vi "ExcelReport.vi"(6 "SN":string="1", 8 "error in":errorcluster caption="错误输入（无错误）", 10 "列首字符串":string[](array[string])=["测试名称", "TestItem ITEM", "通道", "设置参数", "下限值", "上限值", "单位", "测量值", "结果", "测试时间", "备注", "测试项目"], 11 "TestResults":string[][](table)=[["启动测试程序", "CMD", "启动测试程序", "100", "", "", "", "PASS", "PASS", "27.534000", "", "通信", "0"], ["测量电流", "MeaCurrent", "Current", "Differential", "0.65", "1", "A", "0.75051", "PASS", "1.079000", "", "电流", "0"], ["启动蓝牙模块", "CMD", "启动蓝牙模块", "1000", "", "", "Hex", "PASS", "PASS", "1.065000", "", "蓝牙", "0"], ["延时", "Delay", "", "2", "", "", "s", "", "Done", "2.023000", "延时2s", "蓝牙", "0"], ["蓝牙状态查询", "CMD", "蓝牙状态查询", "1000", "0x00", "0x00", "Hex", "0x00", "PASS", "5.294000", "", "蓝牙", "1"], ["打开蓝牙", "CMD", "蓝牙打开", "100", "0x00", "0x00", "Hex", "0x00", "PASS", "0.185000", "", "蓝牙", "0"], ["设置音量20", "CMD", "设置系统音量20", "100", "0x00", "0x00", "Hex", "0x00", "PASS", "0.189000", "", "通信", "0"], ["启动屏幕校准", "CMD", "启动屏幕校准", "100", "", "", "Hex", "PASS", "PASS", "0.189000", "", "屏幕校准", "0"], ["人工校准屏幕", "Check", "屏幕校准", "VisualCheck.vi", "", "", "", "PASS", "PASS", "11.176000", "", "屏幕校准", "0"], ["启动按键测试", "CMD", "启动按键模块", "100", "", "", "Hex", "PASS", "PASS", "0.169000", "", "按键", "0"], ["按键测试", "Check", "按键", "VisualCheck.vi", "", "", "", "PASS", "PASS", "11.933000", "", "按键", "0"], ["退出按键测试", "CMD", "按键模块退出", "100", "", "", "Hex", "PASS", "PASS", "0.171000", "", "按键", "0"], ["DVD仓口灯光", "Check", "DVD灯光蓝色", "VisualCheck.vi", "", "", "", "PASS", "PASS", "4.402000", "", "DVD", "0"], ["入碟", "Check", "放入CD碟", "VisualCheck.vi", "", "", "", "PASS", "PASS", "6.804000", "", "DVD", "0"], ["DVD仓口灯光", "Check", "DVD灯光红色", "VisualCheck.vi", "", "", "", "PASS", "PASS", "2.171000", "", "DVD", "0"], ["打开ILL", "DOAction", "ILL", "1", "", "", "电平", "", "Done", "0.013000", "", "ILL检测", "0"], ["按键灯", "Check", "按键灯亮", "VisualCheck.vi", "", "", "", "PASS", "PASS", "1.676000", "", "按键", "0"], ["读取ILL状态", "CMD", "ILL状态", "100", "0x01", "0x01", "Hex", "0x01", "PASS", "0.170000", "", "ILL检测", "0"], ["关闭ILL", "DOAction", "ILL", "0", "", "", "电平", "", "Done", "0.013000", "", "ILL检测", "0"], ["打开BACK", "DOAction", "BACK", "1", "", "", "电平", "", "Done", "0.013000", "", "倒车检测", "0"], ["倒车视频", "Check", "倒车视频", "VisualCheck.vi", "", "", "", "PASS", "PASS", "1.476000", "", "倒车检测", "0"], ["读取BACK状态", "CMD", "BACK状态", "100", "0x01", "0x01", "Hex", "0x01", "PASS", "0.169000", "", "倒车检测", "0"], ["关闭BACK", "DOAction", "BACK", "0", "", "", "电平", "", "Done", "0.013000", "", "倒车检测", "0"], ["打开BREAK", "DOAction", "BRAKE", "1", "", "", "电平", "", "Done", "0.013000", "", "刹车检测", "0"], ["延时", "Delay", "", "0.5", "", "", "s", "", "Done", "0.512000", "延时500ms", "刹车检测", "0"], ["读取BREAK状态", "CMD", "BRAKE状态", "100", "0x01", "0x01", "Hex", "0x01", "PASS", "0.190000", "", "刹车检测", "0"], ["关闭BREAK", "DOAction", "BRAKE", "0", "", "", "电平", "", "Done", "0.030000", "", "刹车检测", "0"], ["启动方控模块", "CMD", "启动方控模块", "100", "", "", "Hex", "PASS", "PASS", "0.189000", "", "方控", "0"], ["打开方控1输出", "DOAction", "SW1", "1", "", "", "电平", "", "Done", "0.032000", "", "方控", "0"], ["读取方控1电压值", "CMD", "读取SW1电压", "200", "2.2", "2.5", "Hex", "3.26697", "FAIL", "2.297000", "方控1,2~2.2V", "方控", "0"], ["关闭方控1输出", "DOAction", "SW1", "0", "", "", "电平", "", "Done", "0.030000", "", "方控", "0"], ["打开方控2输出", "DOAction", "SW2", "1", "", "", "电平", "", "Done", "0.030000", "", "方控", "0"], ["读取方控1电压值", "CMD", "读取SW2电压", "100", "2.2", "2.5", "Hex", "3.26858", "FAIL", "1.362000", "方控2,2~2.2V", "方控", "0"], ["关闭方控2输出", "DOAction", "SW2", "0", "", "", "电平", "", "Done", "0.030000", "", "方控", "0"], ["获取蓝牙地址", "CMD", "获取蓝牙地址", "500", "0x000000000000", "0xFFFFFFFFFFFF", "Hex", "0x882020202020", "PASS", "2.216000", "", "蓝牙", "1"], ["延时", "Delay", "", "1", "", "", "s", "", "Done", "1.028000", "延时1s", "蓝牙", "0"], ["蓝牙配对", "CMD", "蓝牙配对", "500", "0x00", "0x00", "Hex", "0x00", "PASS", "3.089000", "", "蓝牙", "1"], ["蓝牙状态查询", "CMD", "蓝牙状态查询", "100", "0x06", "0x06", "Hex", "0x06", "PASS", "0.201000", "", "蓝牙", "1"], ["打开喇叭输出", "DOAction", "SPK", "1", "", "", "电平", "", "Done", "0.043000", "", "蓝牙", "0"], ["延时", "Delay", "", "1", "", "", "s", "", "Done", "1.023000", "延时1s", "蓝牙", "0"], ["音频模拟输出", "AOFreq", "AudioSW", "F=1000HZ,A=0.6V", "", "", "频率", "", "Done", "1.230000", "", "蓝牙", "0"], ["采集蓝牙音频输出", "BlueToothAI", "", "", "", "", "", "", "Done", "4.457000", "", "蓝牙", "0"], ["蓝牙音频频率", "Frequency", "", "", "980", "1020", "Hz", "909.76991", "FAIL", "0.025000", "", "蓝牙", "0"], ["蓝牙音频幅度", "RMS", "", "", "0.2", "0.5", "V", "0.00002", "FAIL", "0.013000", "", "蓝牙", "0"], ["蓝牙音频失真度", "BTTHD", "", "", "0", "1", "%", "100.65435", "FAIL", "0.034000", "", "蓝牙", "0"], ["关闭喇叭输出", "DOAction", "SPK", "0", "", "", "电平", "", "Done", "0.012000", "", "蓝牙", "0"], ["关闭音频模拟输出", "AOFreq", "AudioSW", "F=0HZ,A=0V", "", "", "频率", "", "Done", "1.013000", "", "蓝牙", "0"], ["关闭蓝牙", "CMD", "蓝牙关闭", "500", "0x00", "0x00", "Hex", "0x00", "PASS", "1.596000", "", "蓝牙", "0"], ["退出蓝牙模块", "CMD", "蓝牙模块退出", "100", "", "", "Hex", "PASS", "PASS", "0.539000", "", "蓝牙", "0"], ["清除蓝牙设备", "RemoveBTDevices", "", "", "", "", "", "", "Done", "0.656000", "", "", "0"], ["检测SD卡", "CMD", "SD卡状态", "100", "0x01", "0x01", "Hex", "0x01", "PASS", "0.172000", "", "SD卡", "1"], ["启动SD卡模块", "CMD", "启动SD卡模块", "500", "", "", "Hex", "PASS", "PASS", "3.664000", "", "SD卡", "1"], ["SD卡加载状态", "CMD", "SD卡加载状态", "100", "0x02", "0x02", "Hex", "0x02", "PASS", "0.176000", "", "SD卡", "1"], ["SD卡加载时间", "CMD", "SD卡加载时间", "100", "0", "10", "s", "0.00000", "PASS", "0.273000", "0~10s加载时间", "SD卡", "0"], ["播放SD卡音频2", "CMD", "播放SD卡音频2", "100", "0x00", "0x00", "Hex", "0x00", "PASS", "2.141000", "", "SD卡", "0"], ["延时", "Delay", "", "1", "", "", "s", "", "Done", "1.029000", "延时1s", "SD卡", "0"], ["采集FL音频输出", "AIFreq", "FL", "Differential", "", "", "", "", "Done", "1.037000", "", "SD卡", "0"], ["FL频率", "Frequency", "", "", "990", "1010", "Hz", "999.96860", "PASS", "0.034000", "", "SD卡", "0"], ["FL幅度", "RMS", "", "", "0.9", "1.1", "V", "0.96949", "PASS", "0.016000", "", "SD卡", "0"], ["FL失真度", "THD", "", "", "0", "1", "%", "0.35018", "PASS", "0.065000", "", "SD卡", "0"], ["采集FR音频输出", "AIFreq", "FR", "Differential", "", "", "", "", "Done", "1.019000", "", "SD卡", "0"], ["FR频率", "Frequency", "", "", "990", "1010", "Hz", "999.96849", "PASS", "0.025000", "", "SD卡", "0"], ["FR幅度", "RMS", "", "", "0.9", "1.1", "V", "0.98085", "PASS", "0.014000", "", "SD卡", "0"], ["FR失真度", "THD", "", "", "0", "1", "%", "0.33911", "PASS", "0.044000", "", "SD卡", "0"], ["采集RL音频输出", "AIFreq", "RL", "Differential", "", "", "", "", "Done", "1.018000", "", "SD卡", "0"], ["RL频率", "Frequency", "", "", "990", "1010", "Hz", "999.96854", "PASS", "0.023000", "", "SD卡", "0"], ["RL幅度", "RMS", "", "", "0.9", "1.1", "V", "0.93852", "PASS", "0.015000", "", "SD卡", "0"], ["RL失真度", "THD", "", "", "0", "1", "%", "0.34994", "PASS", "0.051000", "", "SD卡", "0"], ["采集RR音频输出", "AIFreq", "RR", "Differential", "", "", "", "", "Done", "1.020000", "", "SD卡", "0"], ["RR频率", "Frequency", "", "", "990", "1010", "Hz", "999.96869", "PASS", "0.026000", "", "SD卡", "0"], ["RR幅度", "RMS", "", "", "0.9", "1.1", "V", "0.93560", "PASS", "0.014000", "", "SD卡", "0"], ["RR失真度", "THD", "", "", "0", "1", "%", "0.35691", "PASS", "0.051000", "", "SD卡", "0"], ["采集FLOUT音频输出", "AIFreq", "FLOUT", "RSE", "", "", "", "", "Done", "1.018000", "", "SD卡", "0"], ["FLOUT频率", "Frequency", "", "", "990", "1010", "Hz", "999.96842", "PASS", "0.023000", "", "SD卡", "0"], ["FLOUT幅度", "RMS", "", "", "0.09", "0.11", "V", "0.04812", "FAIL", "0.014000", "", "SD卡", "0"], ["采集FROUT音频输出", "AIFreq", "FROUT", "RSE", "", "", "", "", "Done", "1.019000", "", "SD卡", "0"], ["FROUT频率", "Frequency", "", "", "990", "1010", "Hz", "999.96823", "PASS", "0.024000", "", "SD卡", "0"], ["FROUT幅度", "RMS", "", "", "0.09", "0.11", "V", "0.04856", "FAIL", "0.014000", "", "SD卡", "0"], ["采集RLOUT音频输出", "AIFreq", "RLOUT", "RSE", "", "", "", "", "Done", "1.020000", "", "SD卡", "0"], ["RLOUT频率", "Frequency", "", "", "990", "1010", "Hz", "999.96809", "PASS", "0.024000", "", "SD卡", "0"], ["RLOUT幅度", "RMS", "", "", "0.09", "0.11", "V", "0.04613", "FAIL", "0.015000", "", "SD卡", "0"], ["采集RROUT音频输出", "AIFreq", "RROUT", "RSE", "", "", "", "", "Done", "1.018000", "", "SD卡", "0"], ["RROUT频率", "Frequency", "", "", "990", "1010", "Hz", "999.96763", "PASS", "0.025000", "", "SD卡", "0"], ["RROUT幅度", "RMS", "", "", "0.09", "0.11", "V", "0.04594", "FAIL", "0.014000", "", "SD卡", "0"], ["播放SD卡音频7", "CMD", "播放SD卡音频7", "100", "0x00", "0x00", "Hex", "0x00", "PASS", "0.425000", "", "SD卡", "0"], ["延时", "Delay", "", "1", "", "", "s", "", "Done", "1.013000", "延时1s", "SD卡", "0"], ["采集FL音频输出", "AIFreq", "FL", "Differential", "", "", "", "", "Done", "1.039000", "", "SD卡", "0"], ["FL信噪比", "SNR", "", "", "45", "", "db", "53.79027", "PASS", "0.015000", "", "SD卡", "0"], ["采集FR音频输出", "AIFreq", "FR", "Differential", "", "", "", "", "Done", "1.019000", "", "SD卡", "0"], ["FR信噪比", "SNR", "", "", "45", "", "db", "53.09428", "PASS", "0.015000", "", "SD卡", "0"], ["采集RL音频输出", "AIFreq", "RL", "Differential", "", "", "", "", "Done", "1.017000", "", "SD卡", "0"], ["RL信噪比", "SNR", "", "", "45", "", "db", "52.88284", "PASS", "0.014000", "", "SD卡", "0"], ["采集RR音频输出", "AIFreq", "RR", "Differential", "", "", "", "", "Done", "1.018000", "", "SD卡", "0"], ["RR信噪比", "SNR", "", "", "45", "", "db", "53.42465", "PASS", "0.013000", "", "SD卡", "0"], ["播放SD卡音频8", "CMD", "播放SD卡音频8", "100", "0x00", "0x00", "Hex", "0x00", "PASS", "0.425000", "", "SD卡", "0"], ["延时", "Delay", "", "1", "", "", "s", "", "Done", "1.013000", "延时1s", "SD卡", "0"], ["采集FL音频输出", "AIsFreq", "CH1=FL,CH2=FR", "Differential", "", "", "", "", "Done", "1.037000", "", "SD卡", "0"], ["FL分离度", "crosstalk", "", "", "45", "", "db", "52.77644", "PASS", "0.036000", "", "SD卡", "0"], ["采集RL音频输出", "AIsFreq", "CH1=RL,CH2=RR", "Differential", "", "", "", "", "Done", "1.020000", "", "SD卡", "0"], ["RL分离度", "crosstalk", "", "", "45", "", "db", "51.94792", "PASS", "0.032000", "", "SD卡", "0"], ["播放SD卡音频10", "CMD", "播放SD卡音频10", "100", "0x00", "0x00", "Hex", "0x00", "PASS", "0.432000", "", "SD卡", "0"], ["延时", "Delay", "", "1", "", "", "s", "", "Done", "1.013000", "延时1s", "SD卡", "0"], ["采集FR音频输出", "AIsFreq", "CH1=FR,CH2=FL", "Differential", "", "", "", "", "Done", "1.037000", "", "SD卡", "0"], ["FR分离度", "crosstalk", "", "", "45", "", "db", "52.76491", "PASS", "0.034000", "", "SD卡", "0"], ["采集RR音频输出", "AIsFreq", "CH1=RR,CH2=RL", "Differential", "", "", "", "", "Done", "1.019000", "", "SD卡", "0"], ["RR分离度", "crosstalk", "", "", "45", "", "db", "51.83152", "PASS", "0.034000", "", "SD卡", "0"], ["退出SD卡模块", "CMD", "SD卡模块退出", "100", "", "", "Hex", "PASS", "PASS", "0.486000", "", "SD卡", "0"], ["检测USB", "CMD", "USB状态", "100", "0x01", "0x01", "Hex", "0x00", "FAIL", "3.035000", "", "USB", "1"], ["启动USB模块", "CMD", "启动USB模块", "500", "", "", "Hex", "", "Skip", "0.032000", "", "USB", "1"], ["USB加载状态", "CMD", "USB加载状态", "100", "0x02", "0x02", "Hex", "", "Skip", "0.020000", "", "USB", "0"], ["USB加载时间", "CMD", "USB加载时间", "100", "0", "10", "s", "", "Skip", "0.012000", "1~10s加载时间", "USB", "0"], ["退出USB模块", "CMD", "USB模块退出", "100", "", "", "Hex", "", "Skip", "0.013000", "", "USB", "0"], ["设置音量20", "CMD", "设置系统音量20", "100", "0x00", "0x00", "Hex", "0x00", "PASS", "0.174000", "", "通信", "0"], ["IPOD_DET下拉", "DOAction", "IPOD_DET", "1", "", "", "电平", "", "Done", "0.015000", "", "IPOD", "0"], ["延时", "Delay", "", "0.5", "", "", "s", "", "Done", "0.514000", "延时0.5s", "IPOD", "0"], ["启动IPOD模块", "CMD", "启动IPOD", "500", "", "", "Hex", "PASS", "PASS", "2.413000", "", "IPOD", "1"], ["IPOD通信测试", "CMD", "IPOD通信自检", "100", "0x00", "0x00", "Hex", "0x00", "PASS", "0.498000", "", "IPOD", "0"], ["打开IPOD电压通道", "DOAction", "DO_IPOD+5V", "1", "", "", "电平", "", "Done", "0.033000", "", "IPOD", "0"], ["IPOD+5V检测", "AIVolt", "IPOD+5V", "", "4.8", "5.5", "V", "5.30354", "PASS", "0.141000", "", "IPOD", "0"], ["关闭IPOD电压通道", "DOAction", "DO_IPOD+5V", "0", "", "", "电平", "", "Done", "0.014000", "", "IPOD", "0"], ["打开IPOD音频通道", "DOAction", "LineOut1", "1", "", "", "电平", "", "Done", "0.015000", "", "IPOD", "0"], ["音频模拟输出", "AOFreq", "AudioSW", "F=1000HZ,A=1V", "", "", "频率", "", "Done", "1.114000", "", "IPOD", "0"], ["采集音频输出", "AIFreq", "FL", "Differential", "", "", "", "", "Done", "1.040000", "", "IPOD", "0"], ["频率", "Frequency", "", "", "990", "1010", "Hz", "1000.00001", "PASS", "0.025000", "", "IPOD", "0"], ["幅度", "RMS", "", "", "0.9", "1.2", "V", "1.06999", "PASS", "0.014000", "", "IPOD", "0"], ["失真度", "THD", "", "", "0", "1", "%", "0.28079", "PASS", "0.047000", "", "IPOD", "0"], ["关闭音频模拟输出", "AOFreq", "AudioSW", "F=0HZ,A=0V", "", "", "频率", "", "Done", "1.015000", "", "IPOD", "0"], ["关闭IPOD音频通道", "DOAction", "LineOut1", "0", "", "", "电平", "", "Done", "0.033000", "", "IPOD", "0"], ["退出IPOD", "CMD", "IPOD退出", "100", "", "", "Hex", "PASS", "PASS", "0.241000", "", "IPOD", "0"], ["启动终端模块", "CMD", "启动TN", "500", "", "", "Hex", "PASS", "PASS", "0.562000", "", "终端", "0"], ["终端通信测试", "CMD", "TN通信自检", "500", "0x00", "0x00", "Hex", "0x00", "PASS", "0.561000", "", "终端", "0"], ["设置TN音量31", "CMD", "设置TN音量31", "100", "0x00", "0x00", "Hex", "0x00", "PASS", "0.166000", "", "终端", "0"], ["打开终端音频通道", "DOAction", "LineOut2", "1", "0x00", "0x00", "电平", "", "Done", "0.004000", "", "终端", "0"], ["音频模拟输出", "AOFreq", "AudioSW", "F=1000HZ,A=1V", "", "", "频率", "", "Done", "1.102000", "", "终端", "0"], ["采集音频输出", "AIFreq", "FL", "Differential", "", "", "", "", "Done", "1.042000", "", "终端", "0"], ["频率", "Frequency", "", "", "990", "1010", "Hz", "1000.00004", "PASS", "0.025000", "", "终端", "0"], ["幅度", "RMS", "", "", "0.9", "1.2", "V", "1.05423", "PASS", "0.017000", "", "终端", "0"], ["失真度", "THD", "", "", "0", "1", "%", "0.31067", "PASS", "0.040000", "", "终端", "0"], ["关闭音频模拟输出", "AOFreq", "AudioSW", "F=0HZ,A=0V", "", "", "频率", "", "Done", "1.014000", "", "终端", "0"], ["关闭终端音频通道", "DOAction", "LineOut2", "0", "", "", "电平", "", "Done", "0.034000", "", "终端", "0"], ["退出终端", "CMD", "TN退出", "100", "", "", "Hex", "PASS", "PASS", "0.183000", "", "终端", "0"], ["启动数字电视模块", "CMD", "启动数字电视", "500", "", "", "Hex", "PASS", "PASS", "6.766000", "", "数字电视", "0"], ["数字电视通信测试", "CMD", "数字电视通信自检", "100", "0x00", "0x00", "Hex", "0x00", "PASS", "0.497000", "", "数字电视", "0"], ["打开DTV音频通道", "DOAction", "LineOut3", "1", "", "", "电平", "", "Done", "0.034000", "", "数字电视", "0"], ["音频模拟输出", "AOFreq", "AudioSW", "F=1000HZ,A=1V", "", "", "频率", "", "Done", "1.119000", "", "数字电视", "0"], ["采集音频输出", "AIFreq", "FL", "Differential", "", "", "", "", "Done", "1.040000", "", "数字电视", "0"], ["频率", "Frequency", "", "", "990", "1010", "Hz", "1000.00015", "PASS", "0.026000", "", "数字电视", "0"], ["幅度", "RMS", "", "", "0.9", "1.2", "V", "1.07136", "PASS", "0.014000", "", "数字电视", "0"], ["失真度", "THD", "", "", "0", "1", "%", "0.31151", "PASS", "0.048000", "", "数字电视", "0"], ["关闭音频模拟输出", "AOFreq", "AudioSW", "F=0HZ,A=0V", "", "", "频率", "", "Done", "1.014000", "", "数字电视", "0"], ["关闭终端音频通道", "DOAction", "LineOut3", "0", "", "", "电平", "", "Done", "0.035000", "", "数字电视", "0"], ["检测视频输出", "Check", "视频播放", "VisualCheck.vi", "", "", "", "PASS", "PASS", "2.188000", "", "数字电视", "0"], ["退出数字电视", "CMD", "数字电视退出", "100", "", "", "Hex", "PASS", "PASS", "0.323000", "", "数字电视", "0"], ["启动AUXIN模块", "CMD", "启动AUXIN", "500", "", "", "Hex", "PASS", "PASS", "3.662000", "", "AuxIn", "0"], ["打开AUXIN音频通道", "DOAction", "LineOut4", "1", "", "", "电平", "", "Done", "0.036000", "", "AuxIn", "0"], ["音频模拟输出", "AOFreq", "AudioSW", "F=1000HZ,A=1V", "", "", "频率", "", "Done", "1.116000", "", "AuxIn", "0"], ["采集音频输出", "AIFreq", "FL", "Differential", "", "", "", "", "Done", "1.040000", "", "AuxIn", "0"], ["频率", "Frequency", "", "", "990", "1010", "Hz", "1000.00011", "PASS", "0.025000", "", "AuxIn", "0"], ["幅度", "RMS", "", "", "0.9", "1.2", "V", "1.04477", "PASS", "0.014000", "", "AuxIn", "0"], ["失真度", "THD", "", "", "0", "1", "%", "0.30972", "PASS", "0.046000", "", "AuxIn", "0"], ["关闭音频模拟输出", "AOFreq", "AudioSW", "F=0HZ,A=0V", "", "", "频率", "", "Done", "1.015000", "", "AuxIn", "0"], ["关闭终端音频通道", "DOAction", "LineOut4", "0", "", "", "电平", "", "Done", "0.036000", "", "AuxIn", "0"], ["检测视频输出", "Check", "视频播放", "VisualCheck.vi", "", "", "", "PASS", "PASS", "1.386000", "", "AuxIn", "0"], ["退出AUXIN", "CMD", "AUXIN退出", "100", "", "", "Hex", "PASS", "PASS", "0.322000", "", "AuxIn", "0"], ["检测DVD状态", "CMD", "DVD碟片状态", "100", "0x01", "0x01", "Hex", "0x01", "PASS", "0.174000", "", "DVD", "1"], ["启动DVD模块", "CMD", "启动DVD模块", "1000", "", "", "", "PASS", "PASS", "2.408000", "", "DVD", "1"], ["等待读碟", "Check", "等待读碟", "VisualCheck.vi", "", "", "", "PASS", "PASS", "14.299000", "", "DVD", "0"], ["DVD加载状态", "CMD", "DVD加载状态", "100", "0x02", "0x02", "Hex", "0x02", "PASS", "0.882000", "", "DVD", "1"], ["DVD加载时间", "CMD", "DVD加载时间", "100", "5", "20", "s", "13.00000", "PASS", "0.198000", "5~20秒加载时间", "DVD", "0"], ["DVD碟片类型", "CMD", "DVD碟片类型", "100", "0x03", "0x03", "Hex", "0x03", "PASS", "1.759000", "CD碟", "DVD", "1"], ["播放DVD曲目2", "CMD", "播放DVD音频2", "100", "0x00", "0x00", "Hex", "0x00", "PASS", "0.548000", "1V 0dB音频", "DVD", "0"], ["延时", "Delay", "", "1", "", "", "s", "", "Done", "1.035000", "延时2s", "DVD", "0"], ["采集FL音频输出", "AIFreq", "FL", "Differential", "", "", "", "", "Done", "1.044000", "", "DVD", "0"], ["FL频率", "Frequency", "", "", "990", "1010", "Hz", "999.96399", "PASS", "0.026000", "", "DVD", "0"], ["FL幅度", "RMS", "", "", "0.9", "1.1", "V", "0.97179", "PASS", "0.016000", "", "DVD", "0"], ["FL失真度", "THD", "", "", "0", "1", "%", "0.61446", "PASS", "0.053000", "", "DVD", "0"], ["采集FR音频输出", "AIFreq", "FR", "Differential", "", "", "", "", "Done", "1.019000", "", "DVD", "0"], ["FR频率", "Frequency", "", "", "990", "1010", "Hz", "999.96393", "PASS", "0.027000", "", "DVD", "0"], ["FR幅度", "RMS", "", "", "0.9", "1.1", "V", "0.98312", "PASS", "0.017000", "", "DVD", "0"], ["FR失真度", "THD", "", "", "0", "1", "%", "0.47579", "PASS", "0.053000", "", "DVD", "0"], ["采集RL音频输出", "AIFreq", "RL", "Differential", "", "", "", "", "Done", "1.018000", "", "DVD", "0"], ["RL频率", "Frequency", "", "", "990", "1010", "Hz", "999.96392", "PASS", "0.026000", "", "DVD", "0"], ["RL幅度", "RMS", "", "", "0.9", "1.1", "V", "0.94066", "PASS", "0.016000", "", "DVD", "0"], ["RL失真度", "THD", "", "", "0", "1", "%", "0.56466", "PASS", "0.052000", "", "DVD", "0"], ["采集RR音频输出", "AIFreq", "RR", "Differential", "", "", "", "", "Done", "1.018000", "", "DVD", "0"], ["RR频率", "Frequency", "", "", "990", "1010", "Hz", "999.96381", "PASS", "0.026000", "", "DVD", "0"], ["RR幅度", "RMS", "", "", "0.9", "1.1", "V", "0.93745", "PASS", "0.016000", "", "DVD", "0"], ["RR失真度", "THD", "", "", "0", "1", "%", "0.50204", "PASS", "0.053000", "", "DVD", "0"], ["采集FLOUT音频输出", "AIFreq", "FLOUT", "RSE", "", "", "", "", "Done", "1.019000", "", "DVD", "0"], ["FLOUT频率", "Frequency", "", "", "990", "1010", "Hz", "999.96370", "PASS", "0.026000", "", "DVD", "0"], ["FLOUT幅度", "RMS", "", "", "0.09", "0.11", "V", "0.04854", "FAIL", "0.016000", "", "DVD", "0"], ["采集FROUT音频输出", "AIFreq", "FROUT", "RSE", "", "", "", "", "Done", "1.022000", "", "DVD", "0"], ["FROUT频率", "Frequency", "", "", "990", "1010", "Hz", "999.96362", "PASS", "0.025000", "", "DVD", "0"], ["FROUT幅度", "RMS", "", "", "0.09", "0.11", "V", "0.04898", "FAIL", "0.016000", "", "DVD", "0"], ["采集RLOUT音频输出", "AIFreq", "RLOUT", "RSE", "", "", "", "", "Done", "1.020000", "", "DVD", "0"], ["RLOUT频率", "Frequency", "", "", "990", "1010", "Hz", "999.96358", "PASS", "0.053000", "", "DVD", "0"], ["RLOUT幅度", "RMS", "", "", "0.09", "0.11", "V", "0.04657", "FAIL", "0.016000", "", "DVD", "0"], ["采集RROUT音频输出", "AIFreq", "RROUT", "RSE", "", "", "", "", "Done", "1.020000", "", "DVD", "0"], ["RROUT频率", "Frequency", "", "", "990", "1010", "Hz", "999.96353", "PASS", "0.025000", "", "DVD", "0"], ["RROUT幅度", "RMS", "", "", "0.09", "0.11", "V", "0.04637", "FAIL", "0.016000", "", "DVD", "0"], ["播放DVD曲目7", "CMD", "播放DVD音频7", "100", "0x00", "0x00", "Hex", "0x00", "PASS", "0.479000", "", "DVD", "0"], ["延时", "Delay", "", "1", "", "", "s", "", "Done", "1.035000", "延时2s", "DVD", "0"], ["采集FL音频输出", "AIFreq", "FL", "Differential", "", "", "", "", "Done", "1.042000", "", "DVD", "0"], ["FL信噪比", "SNR", "", "", "38", "", "db", "47.98901", "PASS", "0.015000", "", "DVD", "0"], ["采集FR音频输出", "AIFreq", "FR", "Differential", "", "", "", "", "Done", "1.019000", "", "DVD", "0"], ["FR信噪比", "SNR", "", "", "38", "", "db", "44.50484", "PASS", "0.016000", "", "DVD", "0"], ["采集RL音频输出", "AIFreq", "RL", "Differential", "", "", "", "", "Done", "1.021000", "", "DVD", "0"], ["RL信噪比", "SNR", "", "", "38", "", "db", "48.16009", "PASS", "0.015000", "", "DVD", "0"], ["采集RR音频输出", "AIFreq", "RR", "Differential", "", "", "", "", "Done", "1.018000", "", "DVD", "0"], ["RR信噪比", "SNR", "", "", "38", "", "db", "46.64013", "PASS", "0.016000", "", "DVD", "0"], ["播放DVD曲目8", "CMD", "播放DVD音频8", "100", "0x00", "0x00", "Hex", "0x00", "PASS", "0.474000", "", "DVD", "0"], ["延时", "Delay", "", "1", "", "", "s", "", "Done", "1.015000", "延时2s", "DVD", "0"], ["采集FL音频输出", "AIsFreq", "CH1=FL,CH2=FR", "Differential", "", "", "", "", "Done", "1.044000", "", "DVD", "0"], ["FL分离度", "crosstalk", "", "", "38", "", "db", "47.10165", "PASS", "0.038000", "", "DVD", "0"], ["采集RL音频输出", "AIsFreq", "CH1=RL,CH2=RR", "Differential", "", "", "", "", "Done", "1.021000", "", "DVD", "0"], ["RL分离度", "crosstalk", "", "", "38", "", "db", "47.09654", "PASS", "0.037000", "", "DVD", "0"], ["播放DVD曲目10", "CMD", "播放DVD音频10", "100", "0x00", "0x00", "Hex", "0x00", "PASS", "0.528000", "", "DVD", "0"], ["延时", "Delay", "", "1", "", "", "s", "", "Done", "1.036000", "延时2s", "DVD", "0"], ["采集FR音频输出", "AIsFreq", "CH1=FR,CH2=FL", "Differential", "", "", "", "", "Done", "1.043000", "", "DVD", "0"], ["FR分离度", "crosstalk", "", "", "38", "", "db", "40.03478", "PASS", "0.036000", "", "DVD", "0"], ["采集RR音频输出", "AIsFreq", "CH1=RR,CH2=RL", "Differential", "", "", "", "", "Done", "1.022000", "", "DVD", "0"], ["RR分离度", "crosstalk", "", "", "38", "", "db", "48.22640", "PASS", "0.037000", "", "DVD", "0"], ["退出DVD模块", "CMD", "DVD模块退出", "500", "", "", "Hex", "PASS", "PASS", "0.575000", "", "DVD", "0"], ["发送退碟指令", "CMD", "出碟", "100", "", "", "Hex", "PASS", "PASS", "0.198000", "", "通信", "0"], ["换DVD碟", "Check", "换碟", "VisualCheck.vi", "", "", "", "PASS", "PASS", "2.524000", "", "DVD", "0"], ["入碟", "Check", "放入DVD碟", "VisualCheck.vi", "", "", "", "PASS", "PASS", "4.899000", "", "DVD", "0"], ["启动DVD模块", "CMD", "启动DVD模块", "500", "", "", "", "PASS", "PASS", "2.235000", "", "DVD", "1"], ["检测DVD状态", "CMD", "DVD碟片状态", "100", "0x01", "0x01", "Hex", "0x01", "PASS", "0.197000", "", "DVD", "1"], ["等待读碟", "Check", "等待读碟", "VisualCheck.vi", "", "", "", "PASS", "PASS", "11.073000", "", "DVD", "0"], ["DVD加载状态", "CMD", "DVD加载状态", "100", "0x02", "0x02", "Hex", "0x02", "PASS", "0.832000", "", "DVD", "1"], ["DVD加载时间", "CMD", "DVD加载时间", "100", "5", "20", "s", "7.00000", "PASS", "0.502000", "5~20秒加载时间", "DVD", "0"], ["DVD碟片类型", "CMD", "DVD碟片类型", "100", "0x01", "0x01", "Hex", "0x04", "FAIL", "2.823000", "DVD碟", "DVD", "1"], ["播放DVD视频", "CMD", "播放DVD视频", "100", "0x00", "0x00", "Hex", "", "Skip", "0.037000", "", "DVD", "0"], ["延时", "Delay", "", "1", "", "", "s", "", "Skip", "0.016000", "延时1s", "DVD", "0"], ["检测视频输出", "Check", "视频播放", "VisualCheck.vi", "", "", "", "", "Skip", "0.016000", "", "DVD", "0"], ["退出DVD模块", "CMD", "DVD模块退出", "500", "", "", "Hex", "", "Skip", "0.015000", "", "DVD", "0"], ["发送退碟指令", "CMD", "出碟", "100", "", "", "Hex", "PASS", "PASS", "0.427000", "", "通信", "0"], ["检测退碟状态", "Check", "出碟", "VisualCheck.vi", "", "", "", "", "Skip", "0.015000", "", "DVD", "0"], ["启动导航模块", "CMD", "启动导航模块", "500", "", "", "Hex", "0x", "FAIL", "5.089000", "", "导航", "1"], ["导航卡状态", "CMD", "导航卡状态", "100", "0x01", "0x01", "Hex", "", "Skip", "0.036000", "检测到卡", "导航", "0"], ["导航定位状态", "CMD", "导航定位状态", "100", "0x01", "0x01", "Hex", "", "Skip", "0.014000", "定位成功", "导航", "0"], ["导航定位时间", "CMD", "导航定位时间", "100", "10", "200", "s", "", "Skip", "0.015000", "定位时间", "导航", "0"], ["导航可见星数", "CMD", "导航可见星数", "100", "3", "32", "个", "", "Skip", "0.014000", "3到32个卫星数", "导航", "0"], ["查看地图版本", "Check", "查看地图版本", "VisualCheck.vi", "", "", "", "", "Skip", "0.016000", "", "导航", "0"], ["退出导航", "CMD", "导航模块退出", "100", "", "", "Hex", "", "Skip", "0.015000", "", "导航", "0"], ["恢复出厂设置", "CMD", "恢复出厂设置", "500", "", "", "Hex", "PASS", "PASS", "0.574000", "", "通信", "0"], ["拔除USB", "Check", "拔除USB", "VisualCheck.vi", "", "", "", "FAIL", "FAIL", "3.131000", "", "", "0"], ["拔除导航卡", "Check", "拔除导航卡", "VisualCheck.vi", "", "", "", "FAIL", "FAIL", "0.791000", "", "", "0"], ["拔除SD卡", "Check", "拔除SD卡", "VisualCheck.vi", "", "", "", "FAIL", "FAIL", "0.623000", "", "", "0"], ["Reset", "Check", "Reset", "VisualCheck.vi", "", "", "", "PASS", "PASS", "0.727000", "", "", "0"]]) -> (0 "error out":errorcluster caption="错误输出")   [LabVIEW 2013]
uses:
  <vilib>/addons/_office/_wordsub.llb/font.ctl
  <vilib>/Utility/NIReport.llb/NI_report.lvclass
  GlobValue.vi
  <vilib>/addons/_office/excel.llb/Excel Easy Table (str).vi
  <vilib>/Utility/NIReport.llb/Append Text Table to Report (wrap).vi
  <vilib>/addons/_office/NI_ReportGenerationToolkit.lvlib
  <vilib>/Utility/NIReport.llb/Excel/NI_Excel.lvclass
panel:
  # "产品名称\t序列号\t测试时间\t测试项目\t初始条件\t测试动作\t评价标准\t步骤 测试结果\t测试条件设置"
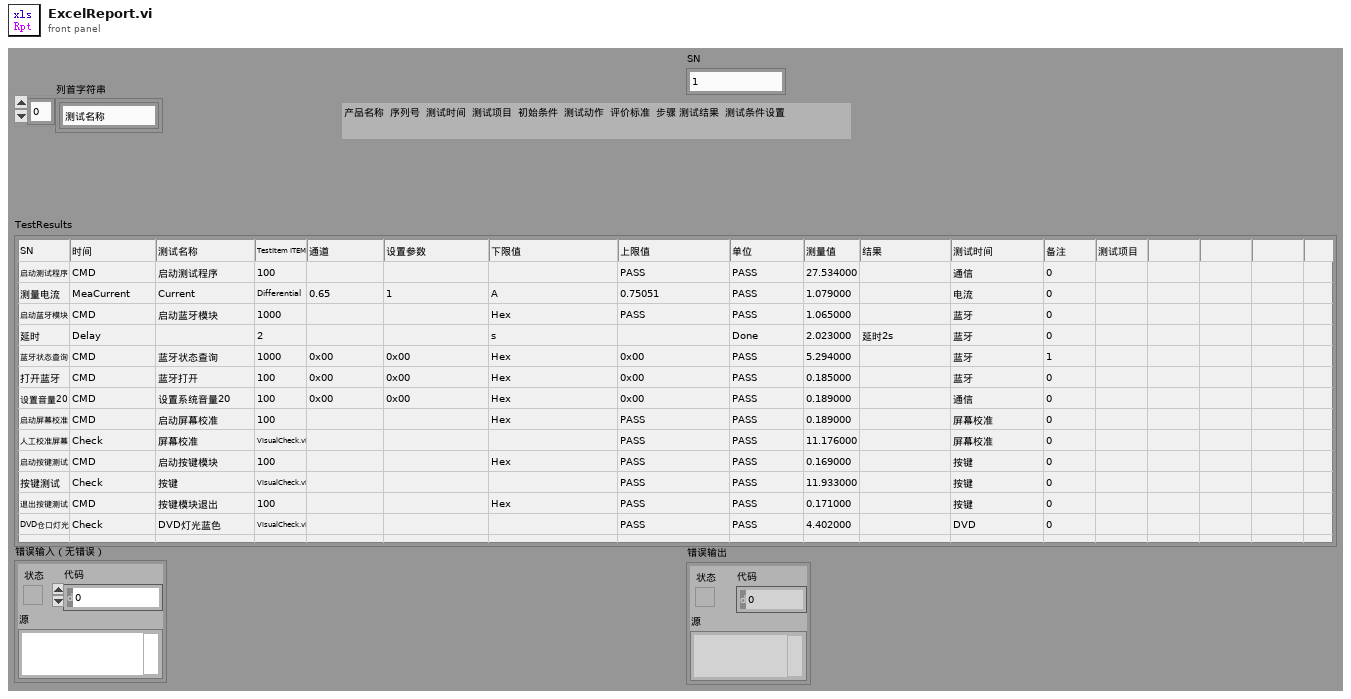
[diagram p1: front panel]
types:
  T1 = typedef "font.ctl" = cluster{"font name":string, "font size":dbl, "bold":u16, "italic":u16, "underline":u16, "strike through":u16, "font color":u32}
  T2 = enum16{"maximized", "minimized", "normal", "no change"}
  T3 = enum16{"Standard Report", "HTML", "Word", "Excel"}
  T4 = cluster{"position (Excel)":cluster{"row":i32, "column":i32}, "name (Excel)":string, "bookmark (Word)":string}
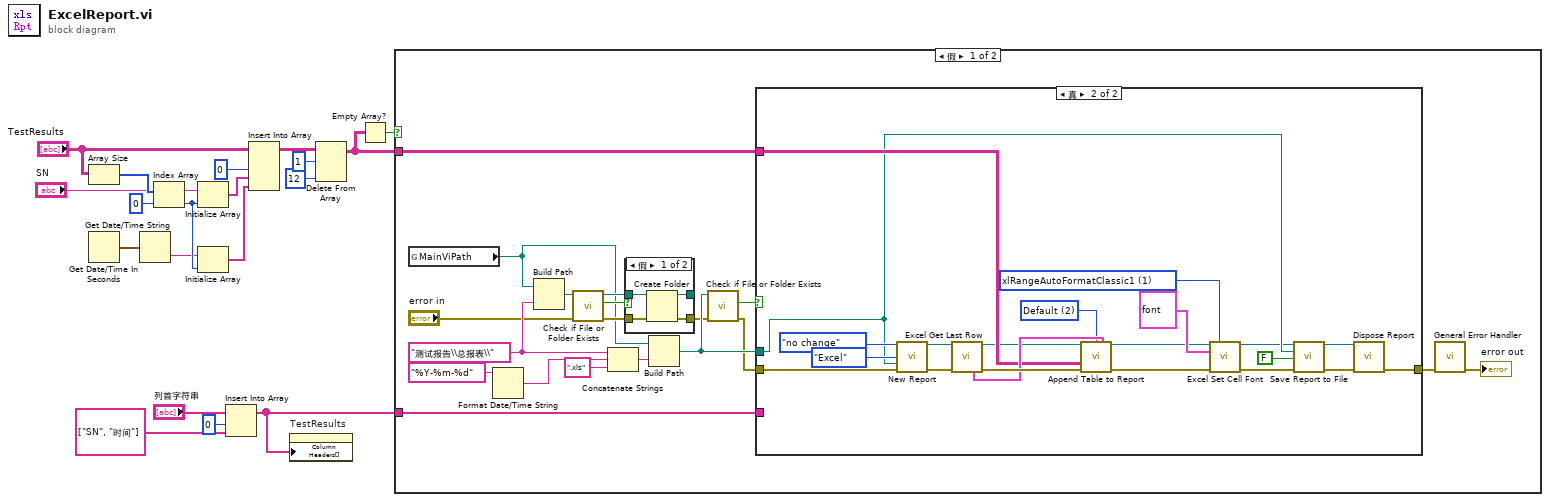
[diagram p0: block diagram]
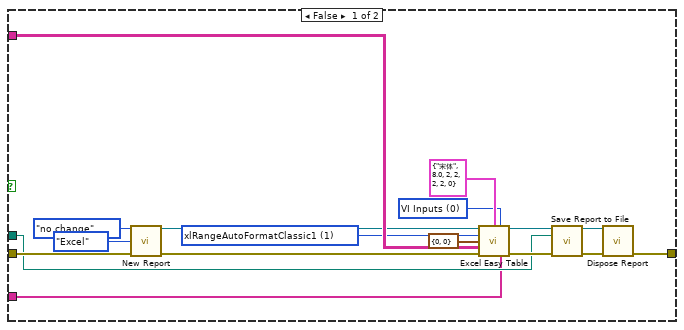
[diagram p3: hidden frame]
diagram:
  n1 = Array Size(array="TestResults") -> (size(s)=w14:i32[])
  n2 = Get Date/Time In Seconds() -> (seconds since 1Jan1904=w11:timestamp)
  n3 = Get Date/Time String(seconds (now)=w11) -> (time string=w9:string)  [unwired: 3 out]
  n4 = Index Array(array=w14, index=0 ("索引")) -> (element=w10:i32)
  n5 = Initialize Array("SN", w10) -> (w12:string[])
  n6 = Initialize Array(w9, w10) -> (w8:string[])
  n7 = Insert Into Array(array="列首字符串", index=0 ("索引"), new element=string[] ["SN", "时间"]) -> (w2:string[])
  n8 = Insert Into Array(array="TestResults", index (col)=0 ("禁用的索引 (列)"), new element #1=w12, new element #2=w8) -> (w7:string[][])  [unwired: 1 in]
  n9 = property on="TestResults" class="Tbl (严格)"("Column Headers[]"=w2) -> ()  [unwired: 2 in, 2 out]
  n10 = Delete From Array(array=w7, length=1 ("长度"), index (col)=12 ("禁用的索引 (列)")) -> (array with subset deleted=w16:string[][])  [unwired: 1 in, 1 out]
  n11 = Empty Array?(array=w16) -> (empty?=w19:bool)
  n12 = case shown="假" w19 {
    tunnel: w16 -> [w33 _]
    tunnel: w2 -> [w31 _]
    frame False {
      w26 = "测试报告\\总报表\\" ("字符串")
      n13 = global read "GlobValue.vi" "MainViPath"() -> (w21:path)
      n14 = Format Date/Time String(time format string (%c)="%Y-%m-%d" ("时间格式字符串(%c)")) -> (date/time string=w23:string)  [unwired: 2 in]
      n15 = Build Path(base path=w21, name or relative path=w26) -> (appended path=w27:path)
      n16 = call <vilib>:"Check if File or Folder Exists.vi"("error in (no error)"="error in", "path"=w27) -> ("error out"=w29:errorcluster, "file or folder exists?"=w28:bool, "dup path"=w30:path)  [unwired: 7 out]
      n17 = Concatenate Strings(w26, w23, ".xls" ("连接的字符串")) -> (w34:string)
      n18 = case shown="假" w28 {
        tunnel: w30 -> [w42 w43]
        tunnel: [w41 _] -> w24
        tunnel: w29 -> [w40 _]
        tunnel: [w39 w43] -> _
        frame False {
          n19 = Create Folder(path (use dialog)=w42, error in=w40) -> (created path=w39:path, error out=w41:errorcluster)  [unwired: 2 out]
        }
        frame True {
        }
      }
      n20 = Build Path(base path=w21, name or relative path=w34) -> (appended path=w38:path)
      n21 = call <vilib>:"Check if File or Folder Exists.vi"("error in (no error)"=w24, "path"=w38) -> ("error out"=w36:errorcluster, "file or folder exists?"=w35:bool)  [unwired: 8 out]
      n22 = case shown="真" w35 {
        tunnel: w36 -> [w59 w80]
        tunnel: w38 -> [w53 w73]
        tunnel: [w56 w79] -> w37
        tunnel: w33 -> [w52 w75]
        tunnel: w31 -> [w44 _]
        frame False {
          w45 = u16 0 items=["VI Inputs", "Font Dialog Box"] ("font settings source")
          w47 = 1 items=["xlRangeAutoFormat3DEffects1"=13, "xlRangeAutoFormat3DEffects2"=14, "xlRangeAutoFormatAccounting1"=4, "xlRangeAutoFormatAccounting2"=5, "xlRangeAutoFormatAccounting3"=6, "xlRangeAutoFormatAccounting4"=17, "xlRangeAutoFormatClassic1"=1, "xlRangeAutoFormatClassic2"=2, "xlRangeAutoFormatClassic3"=3, "xlRangeAutoFormatColor1"=7, "xlRangeAutoFormatColor2"=8, "xlRangeAutoFormatColor3"=9, "xlRangeAutoFormatList1"=10, "xlRangeAutoFormatList2"=11, "xlRangeAutoFormatList3"=12, "xlRangeAutoFormatLocalFormat1"=15, "xlRangeAutoFormatLocalFormat2"=16, "xlRangeAutoFormatLocalFormat3"=19, "xlRangeAutoFormatLocalFormat4"=20, "xlRangeAutoFormatReport1"=21, "xlRangeAutoFormatReport2"=22, "xlRangeAutoFormatReport3"=23, "xlRangeAutoFormatReport4"=24, "xlRangeAutoFormatReport5"=25, "xlRangeAutoFormatReport6"=26, "xlRangeAutoFormatReport7"=27, "xlRangeAutoFormatReport8"=28, "xlRangeAutoFormatReport9"=29, "xlRangeAutoFormatReport10"=30, "xlRangeAutoFormatClassicPivotTable"=31, "xlRangeAutoFormatTable1"=32, "xlRangeAutoFormatTable2"=33, "xlRangeAutoFormatTable3"=34, "xlRangeAutoFormatTable4"=35, "xlRangeAutoFormatTable5"=36, "xlRangeAutoFormatTable6"=37, "xlRangeAutoFormatTable7"=38, "xlRangeAutoFormatTable8"=39, "xlRangeAutoFormatTable9"=40, "xlRangeAutoFormatTable10"=41, "xlRangeAutoFormatPTNone"=42, "xlRangeAutoFormatNone"=-4142, "xlRangeAutoFormatSimple"=-4154] ("auto format")
          n23 = call <vilib>:"New Report.vi"("window state (normal)"=T2."no change", "report type"=T3."Excel", "error in (no error)"=w59) -> ("report out"=w50:refnum<class "NI_report.lvclass">, "error out"=w49:errorcluster)  [unwired: 3 in, 8 out]
          n24 = call-poly <vilib>:"Excel Easy Table.vi"("report in"=w50, "font"=T1 {"font name"="宋体", "font size"=8.0, "bold"=2, "italic"=2, "underline"=2, "strike through"=2, "font color"=0}, "font settings source"=w45, "auto format (none)"=w47, "start (0, 0)"=cluster{"row":i32, "column":i32} {"row"=0, "column"=0} ("position"), "text data"=w52, "error in (no error)"=w49, "column headers"=w44) -> ("report out"=w48:refnum<class "NI_report.lvclass">, "error out"=w55:errorcluster)  [unwired: 3 in, 3 out]
          n25 = call-dynamic "Save Report to File.vi"("report in"=w48, "report file path"=w53, "error in (no error)"=w55) -> ("report out"=w54:refnum<class "NI_report.lvclass">, "error out"=w51:errorcluster)  [unwired: 2 in, 9 out]
          n26 = call-dynamic "Dispose Report.vi"("report in"=w54, "error in (no error)"=w51) -> ("error out"=w56:errorcluster)  [unwired: 13 in]
        }
        frame True {
          w67 = 1 items=["xlRangeAutoFormat3DEffects1"=13, "xlRangeAutoFormat3DEffects2"=14, "xlRangeAutoFormatAccounting1"=4, "xlRangeAutoFormatAccounting2"=5, "xlRangeAutoFormatAccounting3"=6, "xlRangeAutoFormatAccounting4"=17, "xlRangeAutoFormatClassic1"=1, "xlRangeAutoFormatClassic2"=2, "xlRangeAutoFormatClassic3"=3, "xlRangeAutoFormatColor1"=7, "xlRangeAutoFormatColor2"=8, "xlRangeAutoFormatColor3"=9, "xlRangeAutoFormatList1"=10, "xlRangeAutoFormatList2"=11, "xlRangeAutoFormatList3"=12, "xlRangeAutoFormatLocalFormat1"=15, "xlRangeAutoFormatLocalFormat2"=16, "xlRangeAutoFormatLocalFormat3"=19, "xlRangeAutoFormatLocalFormat4"=20, "xlRangeAutoFormatReport1"=21, "xlRangeAutoFormatReport2"=22, "xlRangeAutoFormatReport3"=23, "xlRangeAutoFormatReport4"=24, "xlRangeAutoFormatReport5"=25, "xlRangeAutoFormatReport6"=26, "xlRangeAutoFormatReport7"=27, "xlRangeAutoFormatReport8"=28, "xlRangeAutoFormatReport9"=29, "xlRangeAutoFormatReport10"=30, "xlRangeAutoFormatClassicPivotTable"=31, "xlRangeAutoFormatTable1"=32, "xlRangeAutoFormatTable2"=33, "xlRangeAutoFormatTable3"=34, "xlRangeAutoFormatTable4"=35, "xlRangeAutoFormatTable5"=36, "xlRangeAutoFormatTable6"=37, "xlRangeAutoFormatTable7"=38, "xlRangeAutoFormatTable8"=39, "xlRangeAutoFormatTable9"=40, "xlRangeAutoFormatTable10"=41, "xlRangeAutoFormatPTNone"=42, "xlRangeAutoFormatNone"=-4142, "xlRangeAutoFormatSimple"=-4154] ("auto format")
          w69 = u16 2 items=["US", "Metric", "Default"] ("measurement system")
          n27 = call <vilib>:"New Report.vi"("window state (normal)"=T2."no change", "report type"=T3."Excel", "template (empty)"=w73, "error in (no error)"=w80) -> ("report out"=w70:refnum<class "NI_report.lvclass">, "error out"=w78:errorcluster)  [unwired: 2 in, 8 out]
          n28 = call <vilib>:"Excel Get Last Row.vi"("report in"=w70, "error in (no error)"=w78) -> ("report out"=w66:refnum<class "NI_report.lvclass">, "MS Office parameters out"=w76:T4, "error out"=w77:errorcluster)  [unwired: 1 in, 10 out]
          n29 = call-poly <vilib>:"Append Table to Report.vi"("report in"=w66, "measurement system"=w69, "MS Office parameters"=w76, "text data"=w75, "error in (no error)"=w77) -> ("report out"=w63:refnum<class "NI_report.lvclass">, "error out"=w65:errorcluster)  [unwired: 5 in, 4 out]
          n30 = call <vilib>:"Excel Set Cell Font.vi"("report in"=w63, "auto format"=w67, "font"=T1 {"font name"="Times New Roman", "font size"=10.0, "bold"=2, "italic"=2, "underline"=2, "strike through"=2, "font color"=0}, "error in (no error)"=w65) -> ("report out"=w62:refnum<class "NI_report.lvclass">, "error out"=w64:errorcluster)  [unwired: 10 in]
          n31 = call-dynamic "Save Report to File.vi"("report in"=w62, "report file path"=w73, "prompt to replace? (F)"=FALSE, "error in (no error)"=w64) -> ("report out"=w71:refnum<class "NI_report.lvclass">, "error out"=w72:errorcluster)  [unwired: 1 in, 9 out]
          n32 = call-dynamic "Dispose Report.vi"("report in"=w71, "error in (no error)"=w72) -> ("error out"=w79:errorcluster)  [unwired: 3 in, 10 out]
        }
      }
      n33 = call <vilib>:"General Error Handler.vi"("error in (no error)"=w37) -> ("error out"=→"error out":errorcluster)  [unwired: 10 in, 4 out]
    }
    frame True {
    }
  }
